vi "Measurement Logic.vi"() -> ()   [LabVIEW 2020, in "LPS22Demo.lvlib"]
uses:
  LPS22Demo.lvlib
  Measurement Configuration.ctl
  Measurement Results.ctl
  <vilib>/MeasurementLink/MeasurementLink Measurement Server/Classes/MeasurementContext/MeasurementContext.lvclass
  <instrlib>/niDigital/niDigital.llb/niDigital Data Mapping.ctl
  <instrlib>/niDigital/niDigital.llb/niDigital Bit Order.ctl
  <instrlib>/niDigital/niDigital.llb/niDigital Create Source Waveform (Serial).vi
  <instrlib>/niDigital/niDigital.llb/niDigital Create Capture Waveform (Parallel).vi
  <instrlib>/niDigital/niDigital.llb/niDigital Write Source Waveform (Broadcast U32).vi
  <instrlib>/niDigital/niDigital.llb/niDigital Burst Pattern (Burst Only).vi
  LPS22HH Demo/LPS22HH/LPS22HH.lvlib
panel:
  out "Data":bool[](array[boolean])
  out "R/W":bool=TRUE
  out "Address":bool[](array[boolean])=[FALSE, FALSE, FALSE, TRUE, TRUE, TRUE, TRUE]
  out "Measurement Context out":refnum<class "MeasurementContext.lvclass">
  in  "Measurement Context":refnum<class "MeasurementContext.lvclass">=refnum
  out "Measurement Results":T1={"RX Data"=[1, 0, 1, 1, 0, 0, 1, 1], "Temperature"=0.0, "Error"=""}
  in  "Measurement Configuration":T2={"Open Session"=TRUE, "Close Session "=FALSE, "Register"="WHO_AM_I", "Read/Write"=TRUE, "Write Data"=0} {"Write Data" format="%.0b"}
  out "error out":errorcluster
  in  "error in":errorcluster
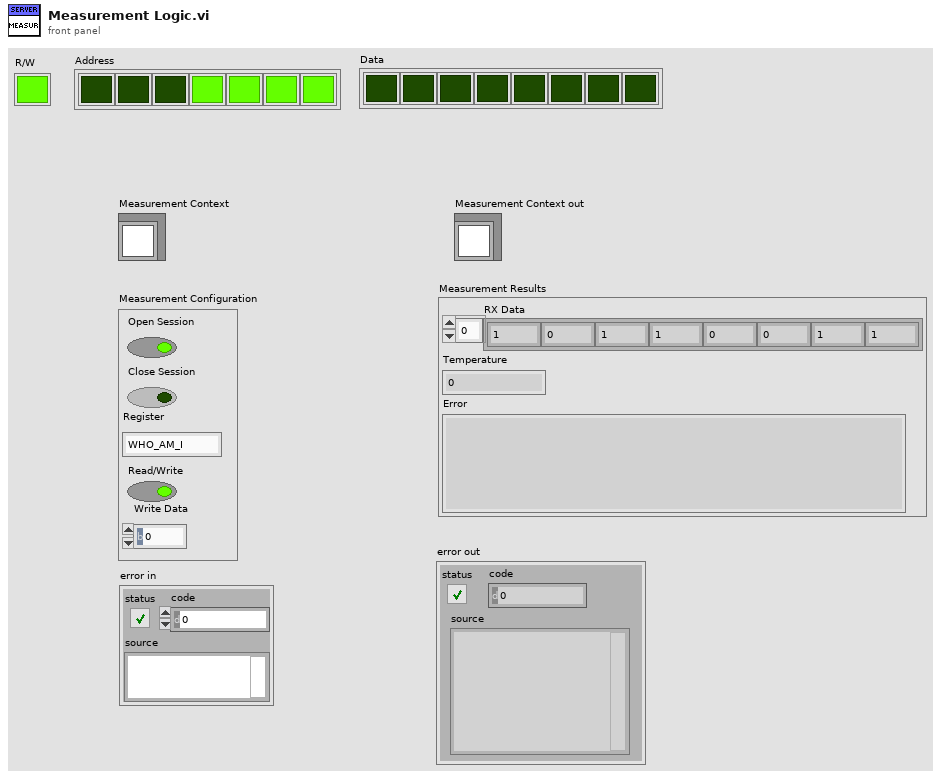
[diagram p1: front panel]
types:
  T1 = typedef "LPS22Demo.lvlib/Measurement Results.ctl" = cluster{"RX Data":u32[], "Temperature":dbl, "Error":string}
  T2 = typedef "LPS22Demo.lvlib/Measurement Configuration.ctl" = cluster{"Open Session":bool, "Close Session ":bool, "Register":string, "Read/Write":bool, "Write Data":i8}
  T3 = typedef "niDigital Bit Order.ctl" = i32
  T4 = typedef "niDigital Data Mapping.ctl" = i32
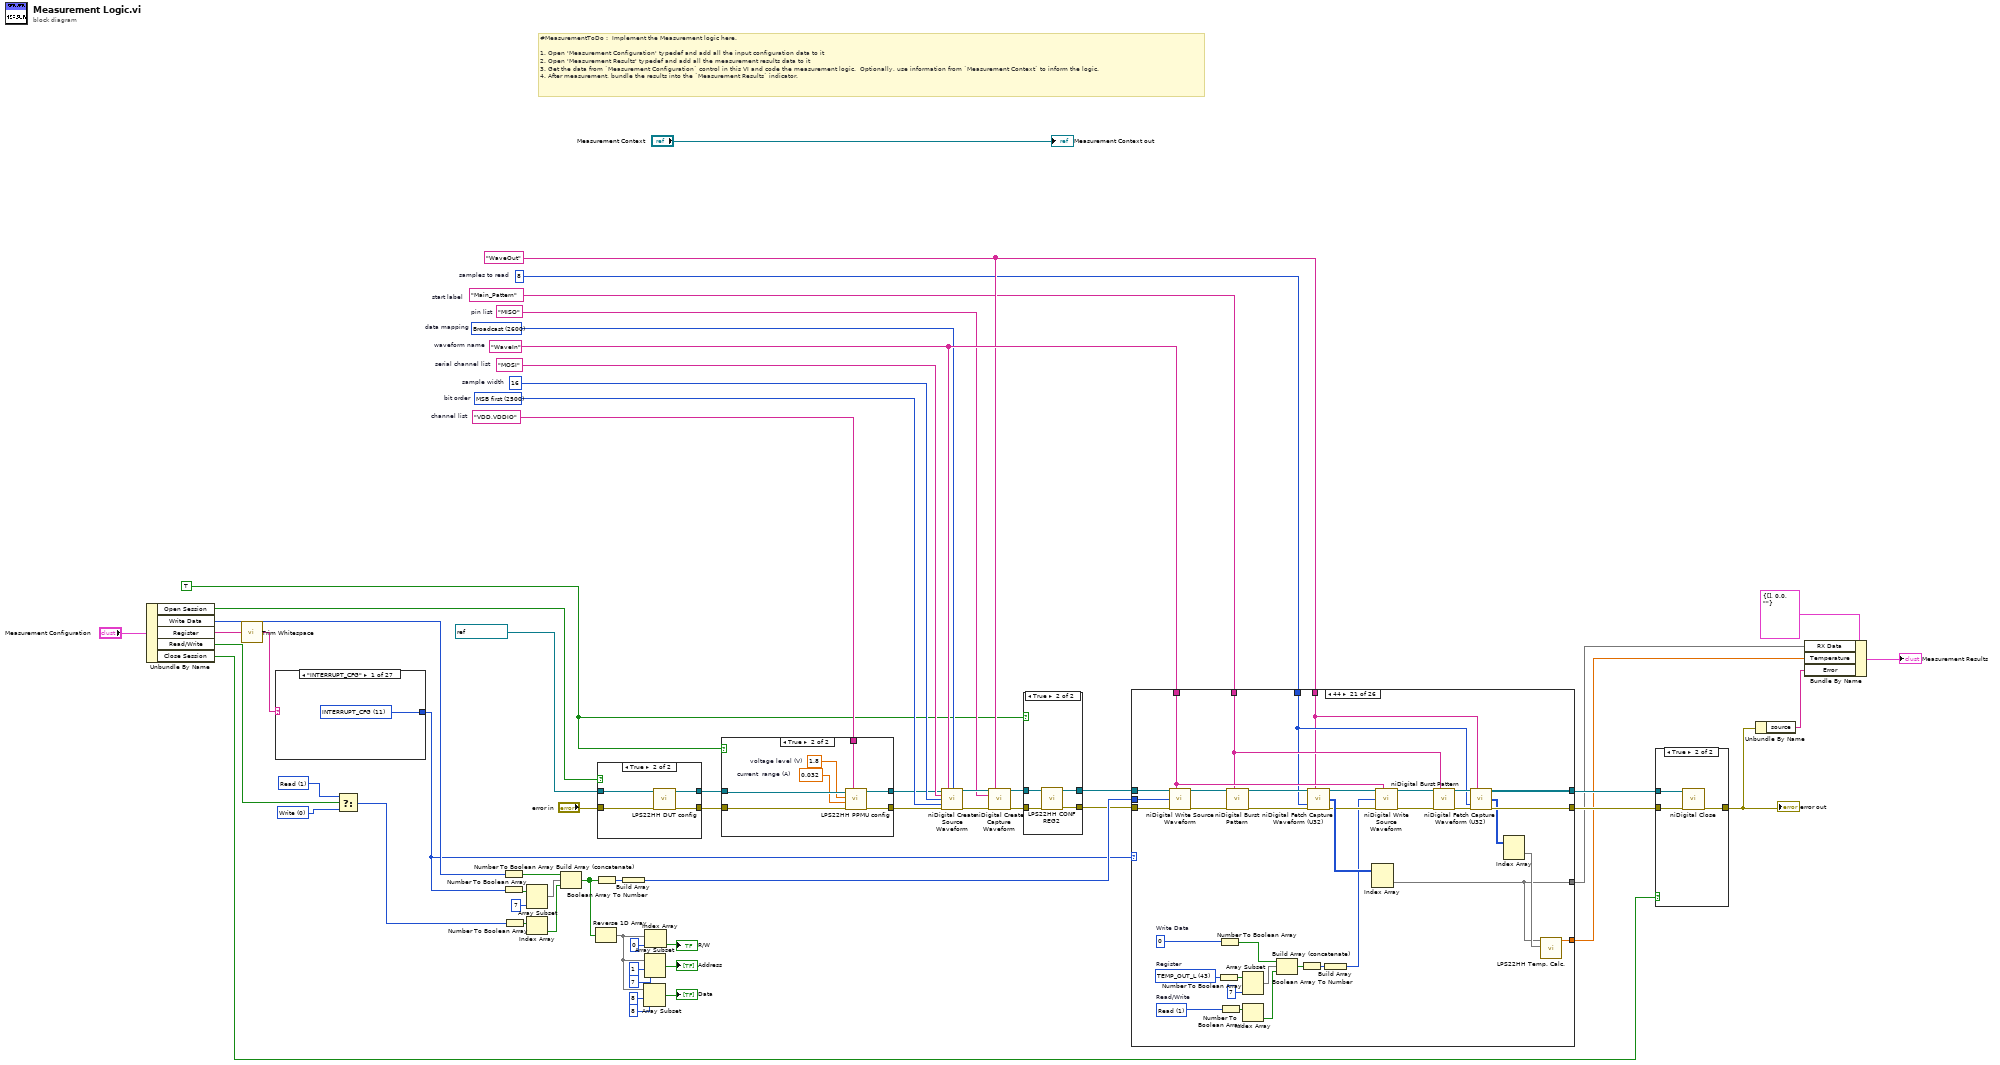
[diagram p0: block diagram]
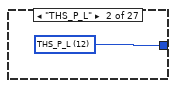
[diagram p2: hidden frame]
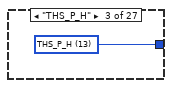
[diagram p3: hidden frame]
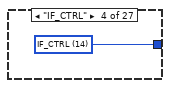
[diagram p4: hidden frame]
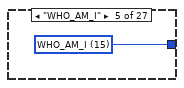
[diagram p5: hidden frame]
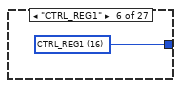
[diagram p6: hidden frame]
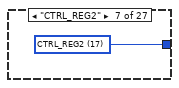
[diagram p7: hidden frame]
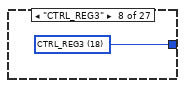
[diagram p8: hidden frame]
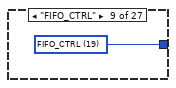
[diagram p9: hidden frame]
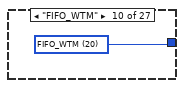
[diagram p10: hidden frame]
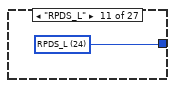
[diagram p11: hidden frame]
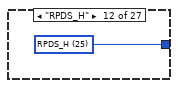
[diagram p12: hidden frame]
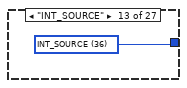
[diagram p13: hidden frame]
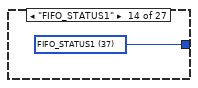
[diagram p14: hidden frame]
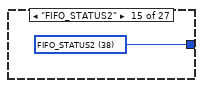
[diagram p15: hidden frame]
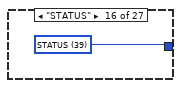
[diagram p16: hidden frame]
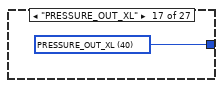
[diagram p17: hidden frame]
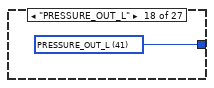
[diagram p18: hidden frame]
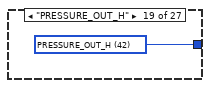
[diagram p19: hidden frame]
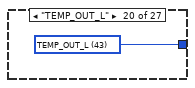
[diagram p20: hidden frame]
diagram:
  w1 = TRUE
  w8 = i16 0 items=["Write", "Read"] ("Read/Write")
  w11 = i16 1 items=["Write", "Read"] ("Read/Write")
  w45 = 8  # samples to read
  w46 = "Main_Pattern"  # start label
  w49 = "VDD,VDDIO"  # channel list
  w53 = "MISO"  # pin list
  w52 = "WaveOut" ("waveform name")
  w59 = "MOSI"  # serial channel list
  w58 = u32 16  # sample width
  w56 = T3 2500 items=["MSB first"=2500, "LSB first"=2501]  # bit order
  w57 = T4 2600 items=["Broadcast"=2600, "Site Unique"=2601]  # data mapping
  w60 = "WaveIn"  # waveform name
  # "#MeasurementToDo :  Implement the Measurement logic here.\n\n1. Open 'Measurement Configuration' typedef and add all the input configuration data to it\n2. Open 'Measurement Results' typedef and add all the measurement results data to it\n3. Get the data from `Measurement Configuration` control in this VI and code the measurement logic.  Optionally, use information from `Measurement Context` to inform the logic.\n4. After measurement, bundle the results into the `Measurement Results` indicator."
  n1 = Unbundle By Name("Measurement Configuration") -> ("Open Session"=w17:bool, "Write Data"=w16:i8, "Register"=w15:string, "Read/Write"=w12:bool, "Close Session"=w9:bool)
  n2 = call <vilib>:"Trim Whitespace.vi"("string"=w15) -> ("trimmed string"=w14:string)  [unwired: 1 in]
  n3 = case shown="\"INTERRUPT_CFG\"" w14 {
    tunnel: [w62 w63 w64 w65 w66 w67 w68 w69 w70 w71 w72 w73 w74 w75 w76 w77 w78 w79 w80 w81 w82 w83 w84 w85 w86 w87 u16 0 ("Register")] -> w13
    frame "INTERRUPT_CFG" {
      w62 = u16 11 items=["INTERRUPT_CFG"=11, "THS_P_L"=12, "THS_P_H"=13, "IF_CTRL"=14, "WHO_AM_I"=15, "CTRL_REG1"=16, "CTRL_REG2"=17, "CTRL_REG3"=18, "FIFO_CTRL"=19, "FIFO_WTM"=20, "RPDS_L"=24, "RPDS_H"=25, "INT_SOURCE"=36, "FIFO_STATUS1"=37, "FIFO_STATUS2"=38, "STATUS"=39, "PRESSURE_OUT_XL"=40, "PRESSURE_OUT_L"=41, "PRESSURE_OUT_H"=42, "TEMP_OUT_L"=43, "TEMP_OUT_H"=44, "FIFO_DATA_OUT_PRESS_XL"=120, "FIFO_DATA_OUT_PRESS_L"=121, "FIFO_DATA_OUT_PRESS_H"=122, "FIFO_DATA_OUT_TEMP_L"=123, "FIFO_DATA_OUT_TEMP_H"=124] ("Register")
    }
    frame "THS_P_L" {
      w63 = u16 12 items=["INTERRUPT_CFG"=11, "THS_P_L"=12, "THS_P_H"=13, "IF_CTRL"=14, "WHO_AM_I"=15, "CTRL_REG1"=16, "CTRL_REG2"=17, "CTRL_REG3"=18, "FIFO_CTRL"=19, "FIFO_WTM"=20, "RPDS_L"=24, "RPDS_H"=25, "INT_SOURCE"=36, "FIFO_STATUS1"=37, "FIFO_STATUS2"=38, "STATUS"=39, "PRESSURE_OUT_XL"=40, "PRESSURE_OUT_L"=41, "PRESSURE_OUT_H"=42, "TEMP_OUT_L"=43, "TEMP_OUT_H"=44, "FIFO_DATA_OUT_PRESS_XL"=120, "FIFO_DATA_OUT_PRESS_L"=121, "FIFO_DATA_OUT_PRESS_H"=122, "FIFO_DATA_OUT_TEMP_L"=123, "FIFO_DATA_OUT_TEMP_H"=124] ("Register")
    }
    frame "THS_P_H" {
      w64 = u16 13 items=["INTERRUPT_CFG"=11, "THS_P_L"=12, "THS_P_H"=13, "IF_CTRL"=14, "WHO_AM_I"=15, "CTRL_REG1"=16, "CTRL_REG2"=17, "CTRL_REG3"=18, "FIFO_CTRL"=19, "FIFO_WTM"=20, "RPDS_L"=24, "RPDS_H"=25, "INT_SOURCE"=36, "FIFO_STATUS1"=37, "FIFO_STATUS2"=38, "STATUS"=39, "PRESSURE_OUT_XL"=40, "PRESSURE_OUT_L"=41, "PRESSURE_OUT_H"=42, "TEMP_OUT_L"=43, "TEMP_OUT_H"=44, "FIFO_DATA_OUT_PRESS_XL"=120, "FIFO_DATA_OUT_PRESS_L"=121, "FIFO_DATA_OUT_PRESS_H"=122, "FIFO_DATA_OUT_TEMP_L"=123, "FIFO_DATA_OUT_TEMP_H"=124] ("Register")
    }
    frame "IF_CTRL" {
      w65 = u16 14 items=["INTERRUPT_CFG"=11, "THS_P_L"=12, "THS_P_H"=13, "IF_CTRL"=14, "WHO_AM_I"=15, "CTRL_REG1"=16, "CTRL_REG2"=17, "CTRL_REG3"=18, "FIFO_CTRL"=19, "FIFO_WTM"=20, "RPDS_L"=24, "RPDS_H"=25, "INT_SOURCE"=36, "FIFO_STATUS1"=37, "FIFO_STATUS2"=38, "STATUS"=39, "PRESSURE_OUT_XL"=40, "PRESSURE_OUT_L"=41, "PRESSURE_OUT_H"=42, "TEMP_OUT_L"=43, "TEMP_OUT_H"=44, "FIFO_DATA_OUT_PRESS_XL"=120, "FIFO_DATA_OUT_PRESS_L"=121, "FIFO_DATA_OUT_PRESS_H"=122, "FIFO_DATA_OUT_TEMP_L"=123, "FIFO_DATA_OUT_TEMP_H"=124] ("Register")
    }
    frame "WHO_AM_I" {
      w66 = u16 15 items=["INTERRUPT_CFG"=11, "THS_P_L"=12, "THS_P_H"=13, "IF_CTRL"=14, "WHO_AM_I"=15, "CTRL_REG1"=16, "CTRL_REG2"=17, "CTRL_REG3"=18, "FIFO_CTRL"=19, "FIFO_WTM"=20, "RPDS_L"=24, "RPDS_H"=25, "INT_SOURCE"=36, "FIFO_STATUS1"=37, "FIFO_STATUS2"=38, "STATUS"=39, "PRESSURE_OUT_XL"=40, "PRESSURE_OUT_L"=41, "PRESSURE_OUT_H"=42, "TEMP_OUT_L"=43, "TEMP_OUT_H"=44, "FIFO_DATA_OUT_PRESS_XL"=120, "FIFO_DATA_OUT_PRESS_L"=121, "FIFO_DATA_OUT_PRESS_H"=122, "FIFO_DATA_OUT_TEMP_L"=123, "FIFO_DATA_OUT_TEMP_H"=124] ("Register")
    }
    frame "CTRL_REG1" {
      w67 = u16 16 items=["INTERRUPT_CFG"=11, "THS_P_L"=12, "THS_P_H"=13, "IF_CTRL"=14, "WHO_AM_I"=15, "CTRL_REG1"=16, "CTRL_REG2"=17, "CTRL_REG3"=18, "FIFO_CTRL"=19, "FIFO_WTM"=20, "RPDS_L"=24, "RPDS_H"=25, "INT_SOURCE"=36, "FIFO_STATUS1"=37, "FIFO_STATUS2"=38, "STATUS"=39, "PRESSURE_OUT_XL"=40, "PRESSURE_OUT_L"=41, "PRESSURE_OUT_H"=42, "TEMP_OUT_L"=43, "TEMP_OUT_H"=44, "FIFO_DATA_OUT_PRESS_XL"=120, "FIFO_DATA_OUT_PRESS_L"=121, "FIFO_DATA_OUT_PRESS_H"=122, "FIFO_DATA_OUT_TEMP_L"=123, "FIFO_DATA_OUT_TEMP_H"=124] ("Register")
    }
    frame "CTRL_REG2" {
      w68 = u16 17 items=["INTERRUPT_CFG"=11, "THS_P_L"=12, "THS_P_H"=13, "IF_CTRL"=14, "WHO_AM_I"=15, "CTRL_REG1"=16, "CTRL_REG2"=17, "CTRL_REG3"=18, "FIFO_CTRL"=19, "FIFO_WTM"=20, "RPDS_L"=24, "RPDS_H"=25, "INT_SOURCE"=36, "FIFO_STATUS1"=37, "FIFO_STATUS2"=38, "STATUS"=39, "PRESSURE_OUT_XL"=40, "PRESSURE_OUT_L"=41, "PRESSURE_OUT_H"=42, "TEMP_OUT_L"=43, "TEMP_OUT_H"=44, "FIFO_DATA_OUT_PRESS_XL"=120, "FIFO_DATA_OUT_PRESS_L"=121, "FIFO_DATA_OUT_PRESS_H"=122, "FIFO_DATA_OUT_TEMP_L"=123, "FIFO_DATA_OUT_TEMP_H"=124] ("Register")
    }
    frame "CTRL_REG3" {
      w69 = u16 18 items=["INTERRUPT_CFG"=11, "THS_P_L"=12, "THS_P_H"=13, "IF_CTRL"=14, "WHO_AM_I"=15, "CTRL_REG1"=16, "CTRL_REG2"=17, "CTRL_REG3"=18, "FIFO_CTRL"=19, "FIFO_WTM"=20, "RPDS_L"=24, "RPDS_H"=25, "INT_SOURCE"=36, "FIFO_STATUS1"=37, "FIFO_STATUS2"=38, "STATUS"=39, "PRESSURE_OUT_XL"=40, "PRESSURE_OUT_L"=41, "PRESSURE_OUT_H"=42, "TEMP_OUT_L"=43, "TEMP_OUT_H"=44, "FIFO_DATA_OUT_PRESS_XL"=120, "FIFO_DATA_OUT_PRESS_L"=121, "FIFO_DATA_OUT_PRESS_H"=122, "FIFO_DATA_OUT_TEMP_L"=123, "FIFO_DATA_OUT_TEMP_H"=124] ("Register")
    }
    frame "FIFO_CTRL" {
      w70 = u16 19 items=["INTERRUPT_CFG"=11, "THS_P_L"=12, "THS_P_H"=13, "IF_CTRL"=14, "WHO_AM_I"=15, "CTRL_REG1"=16, "CTRL_REG2"=17, "CTRL_REG3"=18, "FIFO_CTRL"=19, "FIFO_WTM"=20, "RPDS_L"=24, "RPDS_H"=25, "INT_SOURCE"=36, "FIFO_STATUS1"=37, "FIFO_STATUS2"=38, "STATUS"=39, "PRESSURE_OUT_XL"=40, "PRESSURE_OUT_L"=41, "PRESSURE_OUT_H"=42, "TEMP_OUT_L"=43, "TEMP_OUT_H"=44, "FIFO_DATA_OUT_PRESS_XL"=120, "FIFO_DATA_OUT_PRESS_L"=121, "FIFO_DATA_OUT_PRESS_H"=122, "FIFO_DATA_OUT_TEMP_L"=123, "FIFO_DATA_OUT_TEMP_H"=124] ("Register")
    }
    frame "FIFO_WTM" {
      w71 = u16 20 items=["INTERRUPT_CFG"=11, "THS_P_L"=12, "THS_P_H"=13, "IF_CTRL"=14, "WHO_AM_I"=15, "CTRL_REG1"=16, "CTRL_REG2"=17, "CTRL_REG3"=18, "FIFO_CTRL"=19, "FIFO_WTM"=20, "RPDS_L"=24, "RPDS_H"=25, "INT_SOURCE"=36, "FIFO_STATUS1"=37, "FIFO_STATUS2"=38, "STATUS"=39, "PRESSURE_OUT_XL"=40, "PRESSURE_OUT_L"=41, "PRESSURE_OUT_H"=42, "TEMP_OUT_L"=43, "TEMP_OUT_H"=44, "FIFO_DATA_OUT_PRESS_XL"=120, "FIFO_DATA_OUT_PRESS_L"=121, "FIFO_DATA_OUT_PRESS_H"=122, "FIFO_DATA_OUT_TEMP_L"=123, "FIFO_DATA_OUT_TEMP_H"=124] ("Register")
    }
    frame "RPDS_L" {
      w72 = u16 24 items=["INTERRUPT_CFG"=11, "THS_P_L"=12, "THS_P_H"=13, "IF_CTRL"=14, "WHO_AM_I"=15, "CTRL_REG1"=16, "CTRL_REG2"=17, "CTRL_REG3"=18, "FIFO_CTRL"=19, "FIFO_WTM"=20, "RPDS_L"=24, "RPDS_H"=25, "INT_SOURCE"=36, "FIFO_STATUS1"=37, "FIFO_STATUS2"=38, "STATUS"=39, "PRESSURE_OUT_XL"=40, "PRESSURE_OUT_L"=41, "PRESSURE_OUT_H"=42, "TEMP_OUT_L"=43, "TEMP_OUT_H"=44, "FIFO_DATA_OUT_PRESS_XL"=120, "FIFO_DATA_OUT_PRESS_L"=121, "FIFO_DATA_OUT_PRESS_H"=122, "FIFO_DATA_OUT_TEMP_L"=123, "FIFO_DATA_OUT_TEMP_H"=124] ("Register")
    }
    frame "RPDS_H" {
      w73 = u16 25 items=["INTERRUPT_CFG"=11, "THS_P_L"=12, "THS_P_H"=13, "IF_CTRL"=14, "WHO_AM_I"=15, "CTRL_REG1"=16, "CTRL_REG2"=17, "CTRL_REG3"=18, "FIFO_CTRL"=19, "FIFO_WTM"=20, "RPDS_L"=24, "RPDS_H"=25, "INT_SOURCE"=36, "FIFO_STATUS1"=37, "FIFO_STATUS2"=38, "STATUS"=39, "PRESSURE_OUT_XL"=40, "PRESSURE_OUT_L"=41, "PRESSURE_OUT_H"=42, "TEMP_OUT_L"=43, "TEMP_OUT_H"=44, "FIFO_DATA_OUT_PRESS_XL"=120, "FIFO_DATA_OUT_PRESS_L"=121, "FIFO_DATA_OUT_PRESS_H"=122, "FIFO_DATA_OUT_TEMP_L"=123, "FIFO_DATA_OUT_TEMP_H"=124] ("Register")
    }
    frame "INT_SOURCE" {
      w74 = u16 36 items=["INTERRUPT_CFG"=11, "THS_P_L"=12, "THS_P_H"=13, "IF_CTRL"=14, "WHO_AM_I"=15, "CTRL_REG1"=16, "CTRL_REG2"=17, "CTRL_REG3"=18, "FIFO_CTRL"=19, "FIFO_WTM"=20, "RPDS_L"=24, "RPDS_H"=25, "INT_SOURCE"=36, "FIFO_STATUS1"=37, "FIFO_STATUS2"=38, "STATUS"=39, "PRESSURE_OUT_XL"=40, "PRESSURE_OUT_L"=41, "PRESSURE_OUT_H"=42, "TEMP_OUT_L"=43, "TEMP_OUT_H"=44, "FIFO_DATA_OUT_PRESS_XL"=120, "FIFO_DATA_OUT_PRESS_L"=121, "FIFO_DATA_OUT_PRESS_H"=122, "FIFO_DATA_OUT_TEMP_L"=123, "FIFO_DATA_OUT_TEMP_H"=124] ("Register")
    }
    frame "FIFO_STATUS1" {
      w75 = u16 37 items=["INTERRUPT_CFG"=11, "THS_P_L"=12, "THS_P_H"=13, "IF_CTRL"=14, "WHO_AM_I"=15, "CTRL_REG1"=16, "CTRL_REG2"=17, "CTRL_REG3"=18, "FIFO_CTRL"=19, "FIFO_WTM"=20, "RPDS_L"=24, "RPDS_H"=25, "INT_SOURCE"=36, "FIFO_STATUS1"=37, "FIFO_STATUS2"=38, "STATUS"=39, "PRESSURE_OUT_XL"=40, "PRESSURE_OUT_L"=41, "PRESSURE_OUT_H"=42, "TEMP_OUT_L"=43, "TEMP_OUT_H"=44, "FIFO_DATA_OUT_PRESS_XL"=120, "FIFO_DATA_OUT_PRESS_L"=121, "FIFO_DATA_OUT_PRESS_H"=122, "FIFO_DATA_OUT_TEMP_L"=123, "FIFO_DATA_OUT_TEMP_H"=124] ("Register")
    }
    frame "FIFO_STATUS2" {
      w76 = u16 38 items=["INTERRUPT_CFG"=11, "THS_P_L"=12, "THS_P_H"=13, "IF_CTRL"=14, "WHO_AM_I"=15, "CTRL_REG1"=16, "CTRL_REG2"=17, "CTRL_REG3"=18, "FIFO_CTRL"=19, "FIFO_WTM"=20, "RPDS_L"=24, "RPDS_H"=25, "INT_SOURCE"=36, "FIFO_STATUS1"=37, "FIFO_STATUS2"=38, "STATUS"=39, "PRESSURE_OUT_XL"=40, "PRESSURE_OUT_L"=41, "PRESSURE_OUT_H"=42, "TEMP_OUT_L"=43, "TEMP_OUT_H"=44, "FIFO_DATA_OUT_PRESS_XL"=120, "FIFO_DATA_OUT_PRESS_L"=121, "FIFO_DATA_OUT_PRESS_H"=122, "FIFO_DATA_OUT_TEMP_L"=123, "FIFO_DATA_OUT_TEMP_H"=124] ("Register")
    }
    frame "STATUS" {
      w77 = u16 39 items=["INTERRUPT_CFG"=11, "THS_P_L"=12, "THS_P_H"=13, "IF_CTRL"=14, "WHO_AM_I"=15, "CTRL_REG1"=16, "CTRL_REG2"=17, "CTRL_REG3"=18, "FIFO_CTRL"=19, "FIFO_WTM"=20, "RPDS_L"=24, "RPDS_H"=25, "INT_SOURCE"=36, "FIFO_STATUS1"=37, "FIFO_STATUS2"=38, "STATUS"=39, "PRESSURE_OUT_XL"=40, "PRESSURE_OUT_L"=41, "PRESSURE_OUT_H"=42, "TEMP_OUT_L"=43, "TEMP_OUT_H"=44, "FIFO_DATA_OUT_PRESS_XL"=120, "FIFO_DATA_OUT_PRESS_L"=121, "FIFO_DATA_OUT_PRESS_H"=122, "FIFO_DATA_OUT_TEMP_L"=123, "FIFO_DATA_OUT_TEMP_H"=124] ("Register")
    }
    frame "PRESSURE_OUT_XL" {
      w78 = u16 40 items=["INTERRUPT_CFG"=11, "THS_P_L"=12, "THS_P_H"=13, "IF_CTRL"=14, "WHO_AM_I"=15, "CTRL_REG1"=16, "CTRL_REG2"=17, "CTRL_REG3"=18, "FIFO_CTRL"=19, "FIFO_WTM"=20, "RPDS_L"=24, "RPDS_H"=25, "INT_SOURCE"=36, "FIFO_STATUS1"=37, "FIFO_STATUS2"=38, "STATUS"=39, "PRESSURE_OUT_XL"=40, "PRESSURE_OUT_L"=41, "PRESSURE_OUT_H"=42, "TEMP_OUT_L"=43, "TEMP_OUT_H"=44, "FIFO_DATA_OUT_PRESS_XL"=120, "FIFO_DATA_OUT_PRESS_L"=121, "FIFO_DATA_OUT_PRESS_H"=122, "FIFO_DATA_OUT_TEMP_L"=123, "FIFO_DATA_OUT_TEMP_H"=124] ("Register")
    }
    frame "PRESSURE_OUT_L" {
      w79 = u16 41 items=["INTERRUPT_CFG"=11, "THS_P_L"=12, "THS_P_H"=13, "IF_CTRL"=14, "WHO_AM_I"=15, "CTRL_REG1"=16, "CTRL_REG2"=17, "CTRL_REG3"=18, "FIFO_CTRL"=19, "FIFO_WTM"=20, "RPDS_L"=24, "RPDS_H"=25, "INT_SOURCE"=36, "FIFO_STATUS1"=37, "FIFO_STATUS2"=38, "STATUS"=39, "PRESSURE_OUT_XL"=40, "PRESSURE_OUT_L"=41, "PRESSURE_OUT_H"=42, "TEMP_OUT_L"=43, "TEMP_OUT_H"=44, "FIFO_DATA_OUT_PRESS_XL"=120, "FIFO_DATA_OUT_PRESS_L"=121, "FIFO_DATA_OUT_PRESS_H"=122, "FIFO_DATA_OUT_TEMP_L"=123, "FIFO_DATA_OUT_TEMP_H"=124] ("Register")
    }
    frame "PRESSURE_OUT_H" {
      w80 = u16 42 items=["INTERRUPT_CFG"=11, "THS_P_L"=12, "THS_P_H"=13, "IF_CTRL"=14, "WHO_AM_I"=15, "CTRL_REG1"=16, "CTRL_REG2"=17, "CTRL_REG3"=18, "FIFO_CTRL"=19, "FIFO_WTM"=20, "RPDS_L"=24, "RPDS_H"=25, "INT_SOURCE"=36, "FIFO_STATUS1"=37, "FIFO_STATUS2"=38, "STATUS"=39, "PRESSURE_OUT_XL"=40, "PRESSURE_OUT_L"=41, "PRESSURE_OUT_H"=42, "TEMP_OUT_L"=43, "TEMP_OUT_H"=44, "FIFO_DATA_OUT_PRESS_XL"=120, "FIFO_DATA_OUT_PRESS_L"=121, "FIFO_DATA_OUT_PRESS_H"=122, "FIFO_DATA_OUT_TEMP_L"=123, "FIFO_DATA_OUT_TEMP_H"=124] ("Register")
    }
    frame "TEMP_OUT_L" {
      w81 = u16 43 items=["INTERRUPT_CFG"=11, "THS_P_L"=12, "THS_P_H"=13, "IF_CTRL"=14, "WHO_AM_I"=15, "CTRL_REG1"=16, "CTRL_REG2"=17, "CTRL_REG3"=18, "FIFO_CTRL"=19, "FIFO_WTM"=20, "RPDS_L"=24, "RPDS_H"=25, "INT_SOURCE"=36, "FIFO_STATUS1"=37, "FIFO_STATUS2"=38, "STATUS"=39, "PRESSURE_OUT_XL"=40, "PRESSURE_OUT_L"=41, "PRESSURE_OUT_H"=42, "TEMP_OUT_L"=43, "TEMP_OUT_H"=44, "FIFO_DATA_OUT_PRESS_XL"=120, "FIFO_DATA_OUT_PRESS_L"=121, "FIFO_DATA_OUT_PRESS_H"=122, "FIFO_DATA_OUT_TEMP_L"=123, "FIFO_DATA_OUT_TEMP_H"=124] ("Register")
    }
    frame "TEMP_OUT_H" {
      w82 = u16 44 items=["INTERRUPT_CFG"=11, "THS_P_L"=12, "THS_P_H"=13, "IF_CTRL"=14, "WHO_AM_I"=15, "CTRL_REG1"=16, "CTRL_REG2"=17, "CTRL_REG3"=18, "FIFO_CTRL"=19, "FIFO_WTM"=20, "RPDS_L"=24, "RPDS_H"=25, "INT_SOURCE"=36, "FIFO_STATUS1"=37, "FIFO_STATUS2"=38, "STATUS"=39, "PRESSURE_OUT_XL"=40, "PRESSURE_OUT_L"=41, "PRESSURE_OUT_H"=42, "TEMP_OUT_L"=43, "TEMP_OUT_H"=44, "FIFO_DATA_OUT_PRESS_XL"=120, "FIFO_DATA_OUT_PRESS_L"=121, "FIFO_DATA_OUT_PRESS_H"=122, "FIFO_DATA_OUT_TEMP_L"=123, "FIFO_DATA_OUT_TEMP_H"=124] ("Register")
    }
    frame "FIFO_DATA_OUT_PRESS_XL" {
      w83 = u16 120 items=["INTERRUPT_CFG"=11, "THS_P_L"=12, "THS_P_H"=13, "IF_CTRL"=14, "WHO_AM_I"=15, "CTRL_REG1"=16, "CTRL_REG2"=17, "CTRL_REG3"=18, "FIFO_CTRL"=19, "FIFO_WTM"=20, "RPDS_L"=24, "RPDS_H"=25, "INT_SOURCE"=36, "FIFO_STATUS1"=37, "FIFO_STATUS2"=38, "STATUS"=39, "PRESSURE_OUT_XL"=40, "PRESSURE_OUT_L"=41, "PRESSURE_OUT_H"=42, "TEMP_OUT_L"=43, "TEMP_OUT_H"=44, "FIFO_DATA_OUT_PRESS_XL"=120, "FIFO_DATA_OUT_PRESS_L"=121, "FIFO_DATA_OUT_PRESS_H"=122, "FIFO_DATA_OUT_TEMP_L"=123, "FIFO_DATA_OUT_TEMP_H"=124] ("Register")
    }
    frame "FIFO_DATA_OUT_PRESS_L" {
      w84 = u16 121 items=["INTERRUPT_CFG"=11, "THS_P_L"=12, "THS_P_H"=13, "IF_CTRL"=14, "WHO_AM_I"=15, "CTRL_REG1"=16, "CTRL_REG2"=17, "CTRL_REG3"=18, "FIFO_CTRL"=19, "FIFO_WTM"=20, "RPDS_L"=24, "RPDS_H"=25, "INT_SOURCE"=36, "FIFO_STATUS1"=37, "FIFO_STATUS2"=38, "STATUS"=39, "PRESSURE_OUT_XL"=40, "PRESSURE_OUT_L"=41, "PRESSURE_OUT_H"=42, "TEMP_OUT_L"=43, "TEMP_OUT_H"=44, "FIFO_DATA_OUT_PRESS_XL"=120, "FIFO_DATA_OUT_PRESS_L"=121, "FIFO_DATA_OUT_PRESS_H"=122, "FIFO_DATA_OUT_TEMP_L"=123, "FIFO_DATA_OUT_TEMP_H"=124] ("Register")
    }
    frame "FIFO_DATA_OUT_PRESS_H" {
      w85 = u16 122 items=["INTERRUPT_CFG"=11, "THS_P_L"=12, "THS_P_H"=13, "IF_CTRL"=14, "WHO_AM_I"=15, "CTRL_REG1"=16, "CTRL_REG2"=17, "CTRL_REG3"=18, "FIFO_CTRL"=19, "FIFO_WTM"=20, "RPDS_L"=24, "RPDS_H"=25, "INT_SOURCE"=36, "FIFO_STATUS1"=37, "FIFO_STATUS2"=38, "STATUS"=39, "PRESSURE_OUT_XL"=40, "PRESSURE_OUT_L"=41, "PRESSURE_OUT_H"=42, "TEMP_OUT_L"=43, "TEMP_OUT_H"=44, "FIFO_DATA_OUT_PRESS_XL"=120, "FIFO_DATA_OUT_PRESS_L"=121, "FIFO_DATA_OUT_PRESS_H"=122, "FIFO_DATA_OUT_TEMP_L"=123, "FIFO_DATA_OUT_TEMP_H"=124] ("Register")
    }
    frame "FIFO_DATA_OUT_TEMP_L" {
      w86 = u16 123 items=["INTERRUPT_CFG"=11, "THS_P_L"=12, "THS_P_H"=13, "IF_CTRL"=14, "WHO_AM_I"=15, "CTRL_REG1"=16, "CTRL_REG2"=17, "CTRL_REG3"=18, "FIFO_CTRL"=19, "FIFO_WTM"=20, "RPDS_L"=24, "RPDS_H"=25, "INT_SOURCE"=36, "FIFO_STATUS1"=37, "FIFO_STATUS2"=38, "STATUS"=39, "PRESSURE_OUT_XL"=40, "PRESSURE_OUT_L"=41, "PRESSURE_OUT_H"=42, "TEMP_OUT_L"=43, "TEMP_OUT_H"=44, "FIFO_DATA_OUT_PRESS_XL"=120, "FIFO_DATA_OUT_PRESS_L"=121, "FIFO_DATA_OUT_PRESS_H"=122, "FIFO_DATA_OUT_TEMP_L"=123, "FIFO_DATA_OUT_TEMP_H"=124] ("Register")
    }
    frame "FIFO_DATA_OUT_TEMP_H" {
      w87 = u16 123 items=["INTERRUPT_CFG"=11, "THS_P_L"=12, "THS_P_H"=13, "IF_CTRL"=14, "WHO_AM_I"=15, "CTRL_REG1"=16, "CTRL_REG2"=17, "CTRL_REG3"=18, "FIFO_CTRL"=19, "FIFO_WTM"=20, "RPDS_L"=24, "RPDS_H"=25, "INT_SOURCE"=36, "FIFO_STATUS1"=37, "FIFO_STATUS2"=38, "STATUS"=39, "PRESSURE_OUT_XL"=40, "PRESSURE_OUT_L"=41, "PRESSURE_OUT_H"=42, "TEMP_OUT_L"=43, "TEMP_OUT_H"=44, "FIFO_DATA_OUT_PRESS_XL"=120, "FIFO_DATA_OUT_PRESS_L"=121, "FIFO_DATA_OUT_PRESS_H"=122, "FIFO_DATA_OUT_TEMP_L"=123, "FIFO_DATA_OUT_TEMP_H"=124] ("Register")
    }
    frame "0", Default {
    }
  }
  n4 = Select(t=w11, s=w12, f=w8) -> (s? t:f=w10:i16)
  n5 = Number To Boolean Array(number=w16) -> (Boolean array=w39:bool[])
  n6 = Number To Boolean Array(number=w13) -> (Boolean array=w36:bool[])
  n7 = Number To Boolean Array(number=w10) -> (Boolean array=w35:bool[])
  n8 = Array Subset(array=w36, length=7) -> (w37:bool[])  [unwired: 1 in]
  n9 = Index Array(array=w35) -> (element=w38:bool)  [unwired: 1 in]
  n10 = Build Array (concatenate)(w39, w37, w38) -> (w24:bool[])
  n11 = Reverse 1D Array(array=w24) -> (reversed array=w23:bool[])
  n12 = Boolean Array To Number(Boolean array=w24) -> (number=w40:u32)
  n13 = case shown="True" w17 {
    tunnel: [w90 w94] -> w51
    tunnel: [w89 w93] -> w50
    tunnel: "error in" -> [w89 w92]
    tunnel: refnum<k15> "PBD6571" ("resource name") -> [w90 w91]
    frame False {
    }
    frame True {
      n14 = call "LPS22HH DUT config.vi"("error in"=w92, "resource name"=w91) -> ("error out"=w93:errorcluster, "instrument handle out"=w94:refnum<k15>)  [unwired: 6 in]
    }
  }
  n15 = Build Array(w40) -> (w33:u32[])
  n16 = Array Subset(array=w23, index=8, length=8) -> (→"Data":bool[])
  n17 = Array Subset(array=w23, index=1, length=7) -> (→"Address":bool[])
  n18 = Index Array(array=w23, index=0) -> (element=→"R/W":bool)
  n19 = case shown="True" w1 {
    tunnel: w51 -> [w98 w108]
    tunnel: w50 -> [w100 w107]
    tunnel: w49 -> [w96 w106]
    tunnel: [w97 w104] -> w48
    tunnel: [w99 w103] -> w47
    frame False {
      w95 = 0.032  # current  range (A)
      w101 = 0.0  # voltage level (V)
      n20 = call "LPS22HH PPMU config.vi"("channel list"=w96, "error in"=w100, "current limit range (A)"=w95, "voltage level (V)"=w101, "instrument handle"=w98) -> ("error out"=w99:errorcluster, "instrument handle out"=w97:refnum<k15>)  [unwired: 5 in]
    }
    frame True {
      w102 = 0.032  # current  range (A)
      w105 = 1.8  # voltage level (V)
      n21 = call "LPS22HH PPMU config.vi"("channel list"=w106, "error in"=w107, "current limit range (A)"=w102, "voltage level (V)"=w105, "instrument handle"=w108) -> ("error out"=w103:errorcluster, "instrument handle out"=w104:refnum<k15>)  [unwired: 5 in]
    }
  }
  n22 = call-poly <instrlib>:"niDigital Create Source Waveform.vi"("instrument handle"=w48, "waveform name"=w60, "data mapping"=w57, "pin list"=w59, "sample width"=w58, "bit order"=w56, "error in"=w47) -> ("instrument handle out"=w54:refnum<k15>, "error out"=w55:errorcluster)  [unwired: 7 in]
  n23 = call-poly <instrlib>:"niDigital Create Capture Waveform.vi"("instrument handle"=w54, "waveform name"=w52, "pin list"=w53, "error in"=w55) -> ("instrument handle out"=w42:refnum<k15>, "error out"=w44:errorcluster)  [unwired: 10 in]
  n24 = case shown="True" w1 {
    tunnel: w44 -> [w109 w114]
    tunnel: [w109 w113] -> w22
    tunnel: [w110 w112] -> w43
    tunnel: w42 -> [w110 w111]
    frame False {
    }
    frame True {
      n25 = call "LPS22HH CONF REG2.vi"("error in"=w114, "instrument handle"=w111) -> ("error out"=w113:errorcluster, "instrument handle out"=w112:refnum<k15>)  [unwired: 8 in]
    }
  }
  n26 = case shown="44" w13 {
    tunnel: w60 -> [w122 w146 w162 w178 w194 w210 w226 w242 w258 w274 w290 w306 w322 w338 w354 w370 w386 w402 w418 w426 w462 w506 w522 w538 w554 w570]
    tunnel: w22 -> [w124 w145 w161 w177 w193 w209 w225 w241 w257 w273 w289 w305 w321 w337 w353 w369 w385 w401 w417 w454 w490 w505 w521 w537 w553 w569]
    tunnel: w43 -> [w125 w144 w160 w176 w192 w208 w224 w240 w256 w272 w288 w304 w320 w336 w352 w368 w384 w400 w416 w453 w489 w504 w520 w536 w552 w568]
    tunnel: [w118 w143 w159 w175 w191 w207 w223 w239 w255 w271 w287 w303 w319 w335 w351 w367 w383 w399 w415 w428 w464 w503 w519 w535 w551 w567] -> w41
    tunnel: [w117 w142 w158 w174 w190 w206 w222 w238 w254 w270 w286 w302 w318 w334 w350 w366 w382 w398 w414 w427 w463 w502 w518 w534 w550 w566] -> w21
    tunnel: w52 -> [w119 w141 w157 w173 w189 w205 w221 w237 w253 w269 w285 w301 w317 w333 w349 w365 w381 w397 w413 w423 w459 w501 w517 w533 w549 w565]
    tunnel: w46 -> [w121 w140 w156 w172 w188 w204 w220 w236 w252 w268 w284 w300 w316 w332 w348 w364 w380 w396 w412 w425 w461 w500 w516 w532 w548 w564]
    tunnel: w45 -> [w120 w135 w151 w167 w183 w199 w215 w231 w247 w263 w279 w295 w311 w327 w343 w359 w375 w391 w407 w424 w460 w495 w511 w527 w543 w559]
    tunnel: w33 -> [w123 w133 w149 w165 w181 w197 w213 w229 w245 w261 w277 w293 w309 w325 w341 w357 w373 w389 w405 w447 w483 w493 w509 w525 w541 w557]
    tunnel: [w116 w132 w148 w164 w180 w196 w212 w228 w244 w260 w276 w292 w308 w324 w340 w356 w372 w388 w404 w420 w455 w492 w508 w524 w540 w556] -> w20
    tunnel: [0.0 ("Thermometer") 0.0 ("Thermometer") 0.0 ("Thermometer") 0.0 ("Thermometer") 0.0 ("Thermometer") 0.0 ("Thermometer") 0.0 ("Thermometer") 0.0 ("Thermometer") 0.0 ("Thermometer") 0.0 ("Thermometer") 0.0 ("Thermometer") 0.0 ("Thermometer") 0.0 ("Thermometer") 0.0 ("Thermometer") 0.0 ("Thermometer") 0.0 ("Thermometer") 0.0 ("Thermometer") 0.0 ("Thermometer") 0.0 ("Thermometer") w419 w457 0.0 ("Thermometer") 0.0 ("Thermometer") 0.0 ("Thermometer") 0.0 ("Thermometer") 0.0 ("Thermometer")] -> w19
    frame 11, Default {
      n27 = call-poly <instrlib>:"niDigital Write Source Waveform.vi"("instrument handle"=w125, "waveform name"=w122, "waveform data"=w123, "error in"=w124) -> ("instrument handle out"=w129:refnum<k15>, "error out"=w130:errorcluster)  [unwired: 10 in]
      n28 = call-poly <instrlib>:"niDigital Burst Pattern.vi"("instrument handle"=w129, "start label"=w121, "error in"=w130) -> ("instrument handle out"=w128:refnum<k15>, "error out"=w127:errorcluster)  [unwired: 11 in]
      n29 = call <instrlib>:"niDigital Fetch Capture Waveform (U32).vi"("instrument handle"=w128, "waveform name"=w119, "samples to read"=w120, "error in"=w127) -> ("instrument handle out"=w118:refnum<k15>, "data"=w126:u32[][], "error out"=w117:errorcluster)  [unwired: 9 in]
      n30 = Index Array(array=w126) -> (element=w116:u32[])  [unwired: 2 in]
    }
    frame 12 {
      n31 = call-poly <instrlib>:"niDigital Write Source Waveform.vi"("instrument handle"=w144, "waveform name"=w146, "waveform data"=w133, "error in"=w145) -> ("instrument handle out"=w138:refnum<k15>, "error out"=w139:errorcluster)  [unwired: 10 in]
      n32 = call-poly <instrlib>:"niDigital Burst Pattern.vi"("instrument handle"=w138, "start label"=w140, "error in"=w139) -> ("instrument handle out"=w137:refnum<k15>, "error out"=w136:errorcluster)  [unwired: 11 in]
      n33 = call <instrlib>:"niDigital Fetch Capture Waveform (U32).vi"("instrument handle"=w137, "waveform name"=w141, "samples to read"=w135, "error in"=w136) -> ("instrument handle out"=w143:refnum<k15>, "data"=w134:u32[][], "error out"=w142:errorcluster)  [unwired: 9 in]
      n34 = Index Array(array=w134) -> (element=w132:u32[])  [unwired: 2 in]
    }
    frame 13 {
      n35 = call-poly <instrlib>:"niDigital Write Source Waveform.vi"("instrument handle"=w160, "waveform name"=w162, "waveform data"=w149, "error in"=w161) -> ("instrument handle out"=w154:refnum<k15>, "error out"=w155:errorcluster)  [unwired: 10 in]
      n36 = call-poly <instrlib>:"niDigital Burst Pattern.vi"("instrument handle"=w154, "start label"=w156, "error in"=w155) -> ("instrument handle out"=w153:refnum<k15>, "error out"=w152:errorcluster)  [unwired: 11 in]
      n37 = call <instrlib>:"niDigital Fetch Capture Waveform (U32).vi"("instrument handle"=w153, "waveform name"=w157, "samples to read"=w151, "error in"=w152) -> ("instrument handle out"=w159:refnum<k15>, "data"=w150:u32[][], "error out"=w158:errorcluster)  [unwired: 9 in]
      n38 = Index Array(array=w150) -> (element=w148:u32[])  [unwired: 2 in]
    }
    frame 14 {
      n39 = call-poly <instrlib>:"niDigital Write Source Waveform.vi"("instrument handle"=w176, "waveform name"=w178, "waveform data"=w165, "error in"=w177) -> ("instrument handle out"=w170:refnum<k15>, "error out"=w171:errorcluster)  [unwired: 10 in]
      n40 = call-poly <instrlib>:"niDigital Burst Pattern.vi"("instrument handle"=w170, "start label"=w172, "error in"=w171) -> ("instrument handle out"=w169:refnum<k15>, "error out"=w168:errorcluster)  [unwired: 11 in]
      n41 = call <instrlib>:"niDigital Fetch Capture Waveform (U32).vi"("instrument handle"=w169, "waveform name"=w173, "samples to read"=w167, "error in"=w168) -> ("instrument handle out"=w175:refnum<k15>, "data"=w166:u32[][], "error out"=w174:errorcluster)  [unwired: 9 in]
      n42 = Index Array(array=w166) -> (element=w164:u32[])  [unwired: 2 in]
    }
    frame 15 {
      n43 = call-poly <instrlib>:"niDigital Write Source Waveform.vi"("instrument handle"=w192, "waveform name"=w194, "waveform data"=w181, "error in"=w193) -> ("instrument handle out"=w186:refnum<k15>, "error out"=w187:errorcluster)  [unwired: 10 in]
      n44 = call-poly <instrlib>:"niDigital Burst Pattern.vi"("instrument handle"=w186, "start label"=w188, "error in"=w187) -> ("instrument handle out"=w185:refnum<k15>, "error out"=w184:errorcluster)  [unwired: 11 in]
      n45 = call <instrlib>:"niDigital Fetch Capture Waveform (U32).vi"("instrument handle"=w185, "waveform name"=w189, "samples to read"=w183, "error in"=w184) -> ("instrument handle out"=w191:refnum<k15>, "data"=w182:u32[][], "error out"=w190:errorcluster)  [unwired: 9 in]
      n46 = Index Array(array=w182) -> (element=w180:u32[])  [unwired: 2 in]
    }
    frame 16 {
      n47 = call-poly <instrlib>:"niDigital Write Source Waveform.vi"("instrument handle"=w208, "waveform name"=w210, "waveform data"=w197, "error in"=w209) -> ("instrument handle out"=w202:refnum<k15>, "error out"=w203:errorcluster)  [unwired: 10 in]
      n48 = call-poly <instrlib>:"niDigital Burst Pattern.vi"("instrument handle"=w202, "start label"=w204, "error in"=w203) -> ("instrument handle out"=w201:refnum<k15>, "error out"=w200:errorcluster)  [unwired: 11 in]
      n49 = call <instrlib>:"niDigital Fetch Capture Waveform (U32).vi"("instrument handle"=w201, "waveform name"=w205, "samples to read"=w199, "error in"=w200) -> ("instrument handle out"=w207:refnum<k15>, "data"=w198:u32[][], "error out"=w206:errorcluster)  [unwired: 9 in]
      n50 = Index Array(array=w198) -> (element=w196:u32[])  [unwired: 2 in]
    }
    frame 17 {
      n51 = call-poly <instrlib>:"niDigital Write Source Waveform.vi"("instrument handle"=w224, "waveform name"=w226, "waveform data"=w213, "error in"=w225) -> ("instrument handle out"=w218:refnum<k15>, "error out"=w219:errorcluster)  [unwired: 10 in]
      n52 = call-poly <instrlib>:"niDigital Burst Pattern.vi"("instrument handle"=w218, "start label"=w220, "error in"=w219) -> ("instrument handle out"=w217:refnum<k15>, "error out"=w216:errorcluster)  [unwired: 11 in]
      n53 = call <instrlib>:"niDigital Fetch Capture Waveform (U32).vi"("instrument handle"=w217, "waveform name"=w221, "samples to read"=w215, "error in"=w216) -> ("instrument handle out"=w223:refnum<k15>, "data"=w214:u32[][], "error out"=w222:errorcluster)  [unwired: 9 in]
      n54 = Index Array(array=w214) -> (element=w212:u32[])  [unwired: 2 in]
    }
    frame 18 {
      n55 = call-poly <instrlib>:"niDigital Write Source Waveform.vi"("instrument handle"=w240, "waveform name"=w242, "waveform data"=w229, "error in"=w241) -> ("instrument handle out"=w234:refnum<k15>, "error out"=w235:errorcluster)  [unwired: 10 in]
      n56 = call-poly <instrlib>:"niDigital Burst Pattern.vi"("instrument handle"=w234, "start label"=w236, "error in"=w235) -> ("instrument handle out"=w233:refnum<k15>, "error out"=w232:errorcluster)  [unwired: 11 in]
      n57 = call <instrlib>:"niDigital Fetch Capture Waveform (U32).vi"("instrument handle"=w233, "waveform name"=w237, "samples to read"=w231, "error in"=w232) -> ("instrument handle out"=w239:refnum<k15>, "data"=w230:u32[][], "error out"=w238:errorcluster)  [unwired: 9 in]
      n58 = Index Array(array=w230) -> (element=w228:u32[])  [unwired: 2 in]
    }
    frame 19 {
      n59 = call-poly <instrlib>:"niDigital Write Source Waveform.vi"("instrument handle"=w256, "waveform name"=w258, "waveform data"=w245, "error in"=w257) -> ("instrument handle out"=w250:refnum<k15>, "error out"=w251:errorcluster)  [unwired: 10 in]
      n60 = call-poly <instrlib>:"niDigital Burst Pattern.vi"("instrument handle"=w250, "start label"=w252, "error in"=w251) -> ("instrument handle out"=w249:refnum<k15>, "error out"=w248:errorcluster)  [unwired: 11 in]
      n61 = call <instrlib>:"niDigital Fetch Capture Waveform (U32).vi"("instrument handle"=w249, "waveform name"=w253, "samples to read"=w247, "error in"=w248) -> ("instrument handle out"=w255:refnum<k15>, "data"=w246:u32[][], "error out"=w254:errorcluster)  [unwired: 9 in]
      n62 = Index Array(array=w246) -> (element=w244:u32[])  [unwired: 2 in]
    }
    frame 20 {
      n63 = call-poly <instrlib>:"niDigital Write Source Waveform.vi"("instrument handle"=w272, "waveform name"=w274, "waveform data"=w261, "error in"=w273) -> ("instrument handle out"=w266:refnum<k15>, "error out"=w267:errorcluster)  [unwired: 10 in]
      n64 = call-poly <instrlib>:"niDigital Burst Pattern.vi"("instrument handle"=w266, "start label"=w268, "error in"=w267) -> ("instrument handle out"=w265:refnum<k15>, "error out"=w264:errorcluster)  [unwired: 11 in]
      n65 = call <instrlib>:"niDigital Fetch Capture Waveform (U32).vi"("instrument handle"=w265, "waveform name"=w269, "samples to read"=w263, "error in"=w264) -> ("instrument handle out"=w271:refnum<k15>, "data"=w262:u32[][], "error out"=w270:errorcluster)  [unwired: 9 in]
      n66 = Index Array(array=w262) -> (element=w260:u32[])  [unwired: 2 in]
    }
    frame 24 {
      n67 = call-poly <instrlib>:"niDigital Write Source Waveform.vi"("instrument handle"=w288, "waveform name"=w290, "waveform data"=w277, "error in"=w289) -> ("instrument handle out"=w282:refnum<k15>, "error out"=w283:errorcluster)  [unwired: 10 in]
      n68 = call-poly <instrlib>:"niDigital Burst Pattern.vi"("instrument handle"=w282, "start label"=w284, "error in"=w283) -> ("instrument handle out"=w281:refnum<k15>, "error out"=w280:errorcluster)  [unwired: 11 in]
      n69 = call <instrlib>:"niDigital Fetch Capture Waveform (U32).vi"("instrument handle"=w281, "waveform name"=w285, "samples to read"=w279, "error in"=w280) -> ("instrument handle out"=w287:refnum<k15>, "data"=w278:u32[][], "error out"=w286:errorcluster)  [unwired: 9 in]
      n70 = Index Array(array=w278) -> (element=w276:u32[])  [unwired: 2 in]
    }
    frame 25 {
      n71 = call-poly <instrlib>:"niDigital Write Source Waveform.vi"("instrument handle"=w304, "waveform name"=w306, "waveform data"=w293, "error in"=w305) -> ("instrument handle out"=w298:refnum<k15>, "error out"=w299:errorcluster)  [unwired: 10 in]
      n72 = call-poly <instrlib>:"niDigital Burst Pattern.vi"("instrument handle"=w298, "start label"=w300, "error in"=w299) -> ("instrument handle out"=w297:refnum<k15>, "error out"=w296:errorcluster)  [unwired: 11 in]
      n73 = call <instrlib>:"niDigital Fetch Capture Waveform (U32).vi"("instrument handle"=w297, "waveform name"=w301, "samples to read"=w295, "error in"=w296) -> ("instrument handle out"=w303:refnum<k15>, "data"=w294:u32[][], "error out"=w302:errorcluster)  [unwired: 9 in]
      n74 = Index Array(array=w294) -> (element=w292:u32[])  [unwired: 2 in]
    }
    frame 36 {
      n75 = call-poly <instrlib>:"niDigital Write Source Waveform.vi"("instrument handle"=w320, "waveform name"=w322, "waveform data"=w309, "error in"=w321) -> ("instrument handle out"=w314:refnum<k15>, "error out"=w315:errorcluster)  [unwired: 10 in]
      n76 = call-poly <instrlib>:"niDigital Burst Pattern.vi"("instrument handle"=w314, "start label"=w316, "error in"=w315) -> ("instrument handle out"=w313:refnum<k15>, "error out"=w312:errorcluster)  [unwired: 11 in]
      n77 = call <instrlib>:"niDigital Fetch Capture Waveform (U32).vi"("instrument handle"=w313, "waveform name"=w317, "samples to read"=w311, "error in"=w312) -> ("instrument handle out"=w319:refnum<k15>, "data"=w310:u32[][], "error out"=w318:errorcluster)  [unwired: 9 in]
      n78 = Index Array(array=w310) -> (element=w308:u32[])  [unwired: 2 in]
    }
    frame 37 {
      n79 = call-poly <instrlib>:"niDigital Write Source Waveform.vi"("instrument handle"=w336, "waveform name"=w338, "waveform data"=w325, "error in"=w337) -> ("instrument handle out"=w330:refnum<k15>, "error out"=w331:errorcluster)  [unwired: 10 in]
      n80 = call-poly <instrlib>:"niDigital Burst Pattern.vi"("instrument handle"=w330, "start label"=w332, "error in"=w331) -> ("instrument handle out"=w329:refnum<k15>, "error out"=w328:errorcluster)  [unwired: 11 in]
      n81 = call <instrlib>:"niDigital Fetch Capture Waveform (U32).vi"("instrument handle"=w329, "waveform name"=w333, "samples to read"=w327, "error in"=w328) -> ("instrument handle out"=w335:refnum<k15>, "data"=w326:u32[][], "error out"=w334:errorcluster)  [unwired: 9 in]
      n82 = Index Array(array=w326) -> (element=w324:u32[])  [unwired: 2 in]
    }
    frame 38 {
      n83 = call-poly <instrlib>:"niDigital Write Source Waveform.vi"("instrument handle"=w352, "waveform name"=w354, "waveform data"=w341, "error in"=w353) -> ("instrument handle out"=w346:refnum<k15>, "error out"=w347:errorcluster)  [unwired: 10 in]
      n84 = call-poly <instrlib>:"niDigital Burst Pattern.vi"("instrument handle"=w346, "start label"=w348, "error in"=w347) -> ("instrument handle out"=w345:refnum<k15>, "error out"=w344:errorcluster)  [unwired: 11 in]
      n85 = call <instrlib>:"niDigital Fetch Capture Waveform (U32).vi"("instrument handle"=w345, "waveform name"=w349, "samples to read"=w343, "error in"=w344) -> ("instrument handle out"=w351:refnum<k15>, "data"=w342:u32[][], "error out"=w350:errorcluster)  [unwired: 9 in]
      n86 = Index Array(array=w342) -> (element=w340:u32[])  [unwired: 2 in]
    }
    frame 39 {
      n87 = call-poly <instrlib>:"niDigital Write Source Waveform.vi"("instrument handle"=w368, "waveform name"=w370, "waveform data"=w357, "error in"=w369) -> ("instrument handle out"=w362:refnum<k15>, "error out"=w363:errorcluster)  [unwired: 10 in]
      n88 = call-poly <instrlib>:"niDigital Burst Pattern.vi"("instrument handle"=w362, "start label"=w364, "error in"=w363) -> ("instrument handle out"=w361:refnum<k15>, "error out"=w360:errorcluster)  [unwired: 11 in]
      n89 = call <instrlib>:"niDigital Fetch Capture Waveform (U32).vi"("instrument handle"=w361, "waveform name"=w365, "samples to read"=w359, "error in"=w360) -> ("instrument handle out"=w367:refnum<k15>, "data"=w358:u32[][], "error out"=w366:errorcluster)  [unwired: 9 in]
      n90 = Index Array(array=w358) -> (element=w356:u32[])  [unwired: 2 in]
    }
    frame 40 {
      n91 = call-poly <instrlib>:"niDigital Write Source Waveform.vi"("instrument handle"=w384, "waveform name"=w386, "waveform data"=w373, "error in"=w385) -> ("instrument handle out"=w378:refnum<k15>, "error out"=w379:errorcluster)  [unwired: 10 in]
      n92 = call-poly <instrlib>:"niDigital Burst Pattern.vi"("instrument handle"=w378, "start label"=w380, "error in"=w379) -> ("instrument handle out"=w377:refnum<k15>, "error out"=w376:errorcluster)  [unwired: 11 in]
      n93 = call <instrlib>:"niDigital Fetch Capture Waveform (U32).vi"("instrument handle"=w377, "waveform name"=w381, "samples to read"=w375, "error in"=w376) -> ("instrument handle out"=w383:refnum<k15>, "data"=w374:u32[][], "error out"=w382:errorcluster)  [unwired: 9 in]
      n94 = Index Array(array=w374) -> (element=w372:u32[])  [unwired: 2 in]
    }
    frame 41 {
      n95 = call-poly <instrlib>:"niDigital Write Source Waveform.vi"("instrument handle"=w400, "waveform name"=w402, "waveform data"=w389, "error in"=w401) -> ("instrument handle out"=w394:refnum<k15>, "error out"=w395:errorcluster)  [unwired: 10 in]
      n96 = call-poly <instrlib>:"niDigital Burst Pattern.vi"("instrument handle"=w394, "start label"=w396, "error in"=w395) -> ("instrument handle out"=w393:refnum<k15>, "error out"=w392:errorcluster)  [unwired: 11 in]
      n97 = call <instrlib>:"niDigital Fetch Capture Waveform (U32).vi"("instrument handle"=w393, "waveform name"=w397, "samples to read"=w391, "error in"=w392) -> ("instrument handle out"=w399:refnum<k15>, "data"=w390:u32[][], "error out"=w398:errorcluster)  [unwired: 9 in]
      n98 = Index Array(array=w390) -> (element=w388:u32[])  [unwired: 2 in]
    }
    frame 42 {
      n99 = call-poly <instrlib>:"niDigital Write Source Waveform.vi"("instrument handle"=w416, "waveform name"=w418, "waveform data"=w405, "error in"=w417) -> ("instrument handle out"=w410:refnum<k15>, "error out"=w411:errorcluster)  [unwired: 10 in]
      n100 = call-poly <instrlib>:"niDigital Burst Pattern.vi"("instrument handle"=w410, "start label"=w412, "error in"=w411) -> ("instrument handle out"=w409:refnum<k15>, "error out"=w408:errorcluster)  [unwired: 11 in]
      n101 = call <instrlib>:"niDigital Fetch Capture Waveform (U32).vi"("instrument handle"=w409, "waveform name"=w413, "samples to read"=w407, "error in"=w408) -> ("instrument handle out"=w415:refnum<k15>, "data"=w406:u32[][], "error out"=w414:errorcluster)  [unwired: 9 in]
      n102 = Index Array(array=w406) -> (element=w404:u32[])  [unwired: 2 in]
    }
    frame 43 {
      w432 = i8 0  # Write Data
      w430 = i16 1 items=["Write", "Read"]  # Read/Write
      w431 = u16 44 items=["INTERRUPT_CFG"=11, "THS_P_L"=12, "THS_P_H"=13, "IF_CTRL"=14, "WHO_AM_I"=15, "CTRL_REG1"=16, "CTRL_REG2"=17, "CTRL_REG3"=18, "FIFO_CTRL"=19, "FIFO_WTM"=20, "RPDS_L"=24, "RPDS_H"=25, "INT_SOURCE"=36, "FIFO_STATUS1"=37, "FIFO_STATUS2"=38, "STATUS"=39, "PRESSURE_OUT_XL"=40, "PRESSURE_OUT_L"=41, "PRESSURE_OUT_H"=42, "TEMP_OUT_L"=43, "TEMP_OUT_H"=44, "FIFO_DATA_OUT_PRESS_XL"=120, "FIFO_DATA_OUT_PRESS_L"=121, "FIFO_DATA_OUT_PRESS_H"=122, "FIFO_DATA_OUT_TEMP_L"=123, "FIFO_DATA_OUT_TEMP_H"=124]  # Register
      n103 = call-poly <instrlib>:"niDigital Write Source Waveform.vi"("instrument handle"=w453, "waveform name"=w426, "waveform data"=w447, "error in"=w454) -> ("instrument handle out"=w451:refnum<k15>, "error out"=w452:errorcluster)  [unwired: 10 in]
      n104 = Number To Boolean Array(number=w431) -> (Boolean array=w438:bool[])
      n105 = Number To Boolean Array(number=w432) -> (Boolean array=w435:bool[])
      n106 = Number To Boolean Array(number=w430) -> (Boolean array=w439:bool[])
      n107 = call-poly <instrlib>:"niDigital Burst Pattern.vi"("instrument handle"=w451, "start label"=w425, "error in"=w452) -> ("instrument handle out"=w450:refnum<k15>, "error out"=w449:errorcluster)  [unwired: 11 in]
      n108 = Array Subset(array=w438, length=7) -> (w437:bool[])  [unwired: 1 in]
      n109 = Index Array(array=w439) -> (element=w436:bool)  [unwired: 1 in]
      n110 = Build Array (concatenate)(w435, w437, w436) -> (w440:bool[])
      n111 = Boolean Array To Number(Boolean array=w440) -> (number=w434:u32)
      n112 = call <instrlib>:"niDigital Fetch Capture Waveform (U32).vi"("instrument handle"=w450, "waveform name"=w423, "samples to read"=w424, "error in"=w449) -> ("instrument handle out"=w441:refnum<k15>, "data"=w448:u32[][], "error out"=w442:errorcluster)  [unwired: 9 in]
      n113 = Build Array(w434) -> (w429:u32[])
      n114 = Index Array(array=w448) -> (element=w420:u32[])  [unwired: 2 in]
      n115 = call-poly <instrlib>:"niDigital Write Source Waveform.vi"("instrument handle"=w441, "waveform name"=w426, "waveform data"=w429, "error in"=w442) -> ("instrument handle out"=w445:refnum<k15>, "error out"=w446:errorcluster)  [unwired: 10 in]
      n116 = call-poly <instrlib>:"niDigital Burst Pattern.vi"("instrument handle"=w445, "start label"=w425, "error in"=w446) -> ("instrument handle out"=w444:refnum<k15>, "error out"=w443:errorcluster)  [unwired: 11 in]
      n117 = call <instrlib>:"niDigital Fetch Capture Waveform (U32).vi"("instrument handle"=w444, "waveform name"=w423, "samples to read"=w424, "error in"=w443) -> ("instrument handle out"=w428:refnum<k15>, "data"=w422:u32[][], "error out"=w427:errorcluster)  [unwired: 9 in]
      n118 = Index Array(array=w422) -> (element=w421:u32[])  [unwired: 2 in]
      n119 = call "LPS22HH Temp. Calc..vi"("TEMP_OUT_L"=w420, "TEMP_OUT_H"=w421) -> ("Thermometer"=w419:dbl)  [unwired: 9 in]
    }
    frame 44 {
      w468 = i8 0  # Write Data
      w466 = i16 1 items=["Write", "Read"]  # Read/Write
      w467 = u16 43 items=["INTERRUPT_CFG"=11, "THS_P_L"=12, "THS_P_H"=13, "IF_CTRL"=14, "WHO_AM_I"=15, "CTRL_REG1"=16, "CTRL_REG2"=17, "CTRL_REG3"=18, "FIFO_CTRL"=19, "FIFO_WTM"=20, "RPDS_L"=24, "RPDS_H"=25, "INT_SOURCE"=36, "FIFO_STATUS1"=37, "FIFO_STATUS2"=38, "STATUS"=39, "PRESSURE_OUT_XL"=40, "PRESSURE_OUT_L"=41, "PRESSURE_OUT_H"=42, "TEMP_OUT_L"=43, "TEMP_OUT_H"=44, "FIFO_DATA_OUT_PRESS_XL"=120, "FIFO_DATA_OUT_PRESS_L"=121, "FIFO_DATA_OUT_PRESS_H"=122, "FIFO_DATA_OUT_TEMP_L"=123, "FIFO_DATA_OUT_TEMP_H"=124]  # Register
      n120 = call-poly <instrlib>:"niDigital Write Source Waveform.vi"("instrument handle"=w489, "waveform name"=w462, "waveform data"=w483, "error in"=w490) -> ("instrument handle out"=w487:refnum<k15>, "error out"=w488:errorcluster)  [unwired: 10 in]
      n121 = Number To Boolean Array(number=w467) -> (Boolean array=w474:bool[])
      n122 = Number To Boolean Array(number=w468) -> (Boolean array=w471:bool[])
      n123 = Number To Boolean Array(number=w466) -> (Boolean array=w475:bool[])
      n124 = call-poly <instrlib>:"niDigital Burst Pattern.vi"("instrument handle"=w487, "start label"=w461, "error in"=w488) -> ("instrument handle out"=w486:refnum<k15>, "error out"=w485:errorcluster)  [unwired: 11 in]
      n125 = Array Subset(array=w474, length=7) -> (w473:bool[])  [unwired: 1 in]
      n126 = Index Array(array=w475) -> (element=w472:bool)  [unwired: 1 in]
      n127 = Build Array (concatenate)(w471, w473, w472) -> (w476:bool[])
      n128 = Boolean Array To Number(Boolean array=w476) -> (number=w470:u32)
      n129 = call <instrlib>:"niDigital Fetch Capture Waveform (U32).vi"("instrument handle"=w486, "waveform name"=w459, "samples to read"=w460, "error in"=w485) -> ("instrument handle out"=w477:refnum<k15>, "data"=w484:u32[][], "error out"=w478:errorcluster)  [unwired: 9 in]
      n130 = Build Array(w470) -> (w465:u32[])
      n131 = Index Array(array=w484) -> (element=w455:u32[])  [unwired: 2 in]
      n132 = call-poly <instrlib>:"niDigital Write Source Waveform.vi"("instrument handle"=w477, "waveform name"=w462, "waveform data"=w465, "error in"=w478) -> ("instrument handle out"=w481:refnum<k15>, "error out"=w482:errorcluster)  [unwired: 10 in]
      n133 = call-poly <instrlib>:"niDigital Burst Pattern.vi"("instrument handle"=w481, "start label"=w461, "error in"=w482) -> ("instrument handle out"=w480:refnum<k15>, "error out"=w479:errorcluster)  [unwired: 11 in]
      n134 = call <instrlib>:"niDigital Fetch Capture Waveform (U32).vi"("instrument handle"=w480, "waveform name"=w459, "samples to read"=w460, "error in"=w479) -> ("instrument handle out"=w464:refnum<k15>, "data"=w458:u32[][], "error out"=w463:errorcluster)  [unwired: 9 in]
      n135 = Index Array(array=w458) -> (element=w456:u32[])  [unwired: 2 in]
      n136 = call "LPS22HH Temp. Calc..vi"("TEMP_OUT_L"=w456, "TEMP_OUT_H"=w455) -> ("Thermometer"=w457:dbl)  [unwired: 9 in]
    }
    frame 120 {
      n137 = call-poly <instrlib>:"niDigital Write Source Waveform.vi"("instrument handle"=w504, "waveform name"=w506, "waveform data"=w493, "error in"=w505) -> ("instrument handle out"=w498:refnum<k15>, "error out"=w499:errorcluster)  [unwired: 10 in]
      n138 = call-poly <instrlib>:"niDigital Burst Pattern.vi"("instrument handle"=w498, "start label"=w500, "error in"=w499) -> ("instrument handle out"=w497:refnum<k15>, "error out"=w496:errorcluster)  [unwired: 11 in]
      n139 = call <instrlib>:"niDigital Fetch Capture Waveform (U32).vi"("instrument handle"=w497, "waveform name"=w501, "samples to read"=w495, "error in"=w496) -> ("instrument handle out"=w503:refnum<k15>, "data"=w494:u32[][], "error out"=w502:errorcluster)  [unwired: 9 in]
      n140 = Index Array(array=w494) -> (element=w492:u32[])  [unwired: 2 in]
    }
    frame 121 {
      n141 = call-poly <instrlib>:"niDigital Write Source Waveform.vi"("instrument handle"=w520, "waveform name"=w522, "waveform data"=w509, "error in"=w521) -> ("instrument handle out"=w514:refnum<k15>, "error out"=w515:errorcluster)  [unwired: 10 in]
      n142 = call-poly <instrlib>:"niDigital Burst Pattern.vi"("instrument handle"=w514, "start label"=w516, "error in"=w515) -> ("instrument handle out"=w513:refnum<k15>, "error out"=w512:errorcluster)  [unwired: 11 in]
      n143 = call <instrlib>:"niDigital Fetch Capture Waveform (U32).vi"("instrument handle"=w513, "waveform name"=w517, "samples to read"=w511, "error in"=w512) -> ("instrument handle out"=w519:refnum<k15>, "data"=w510:u32[][], "error out"=w518:errorcluster)  [unwired: 9 in]
      n144 = Index Array(array=w510) -> (element=w508:u32[])  [unwired: 2 in]
    }
    frame 122 {
      n145 = call-poly <instrlib>:"niDigital Write Source Waveform.vi"("instrument handle"=w536, "waveform name"=w538, "waveform data"=w525, "error in"=w537) -> ("instrument handle out"=w530:refnum<k15>, "error out"=w531:errorcluster)  [unwired: 10 in]
      n146 = call-poly <instrlib>:"niDigital Burst Pattern.vi"("instrument handle"=w530, "start label"=w532, "error in"=w531) -> ("instrument handle out"=w529:refnum<k15>, "error out"=w528:errorcluster)  [unwired: 11 in]
      n147 = call <instrlib>:"niDigital Fetch Capture Waveform (U32).vi"("instrument handle"=w529, "waveform name"=w533, "samples to read"=w527, "error in"=w528) -> ("instrument handle out"=w535:refnum<k15>, "data"=w526:u32[][], "error out"=w534:errorcluster)  [unwired: 9 in]
      n148 = Index Array(array=w526) -> (element=w524:u32[])  [unwired: 2 in]
    }
    frame 123 {
      n149 = call-poly <instrlib>:"niDigital Write Source Waveform.vi"("instrument handle"=w552, "waveform name"=w554, "waveform data"=w541, "error in"=w553) -> ("instrument handle out"=w546:refnum<k15>, "error out"=w547:errorcluster)  [unwired: 10 in]
      n150 = call-poly <instrlib>:"niDigital Burst Pattern.vi"("instrument handle"=w546, "start label"=w548, "error in"=w547) -> ("instrument handle out"=w545:refnum<k15>, "error out"=w544:errorcluster)  [unwired: 11 in]
      n151 = call <instrlib>:"niDigital Fetch Capture Waveform (U32).vi"("instrument handle"=w545, "waveform name"=w549, "samples to read"=w543, "error in"=w544) -> ("instrument handle out"=w551:refnum<k15>, "data"=w542:u32[][], "error out"=w550:errorcluster)  [unwired: 9 in]
      n152 = Index Array(array=w542) -> (element=w540:u32[])  [unwired: 2 in]
    }
    frame 124 {
      n153 = call-poly <instrlib>:"niDigital Write Source Waveform.vi"("instrument handle"=w568, "waveform name"=w570, "waveform data"=w557, "error in"=w569) -> ("instrument handle out"=w562:refnum<k15>, "error out"=w563:errorcluster)  [unwired: 10 in]
      n154 = call-poly <instrlib>:"niDigital Burst Pattern.vi"("instrument handle"=w562, "start label"=w564, "error in"=w563) -> ("instrument handle out"=w561:refnum<k15>, "error out"=w560:errorcluster)  [unwired: 11 in]
      n155 = call <instrlib>:"niDigital Fetch Capture Waveform (U32).vi"("instrument handle"=w561, "waveform name"=w565, "samples to read"=w559, "error in"=w560) -> ("instrument handle out"=w567:refnum<k15>, "data"=w558:u32[][], "error out"=w566:errorcluster)  [unwired: 9 in]
      n156 = Index Array(array=w558) -> (element=w556:u32[])  [unwired: 2 in]
    }
  }
  n157 = case shown="True" w9 {
    tunnel: [w571 w574] -> w3
    tunnel: w41 -> [_ w573]
    tunnel: w21 -> [w571 w572]
    frame False {
    }
    frame True {
      n158 = call <instrlib>:"niDigital Close.vi"("instrument handle"=w573, "error in"=w572) -> ("error out"=w574:errorcluster)  [unwired: 13 in]
    }
  }
  "error out" <- w3
  n159 = Unbundle By Name(w3) -> ("source"=w2:string)
  n160 = Bundle By Name(cluster=T1 {"RX Data"=[], "Temperature"=0.0, "Error"=""} ("Measurement Results 2"), "RX Data"=w20, "Temperature"=w19, "Error"=w2) -> (→"Measurement Results":T1)
  "Measurement Context out" <- "Measurement Context"
